vi "Queue_Driver.vi"   [LabVIEW 2023]
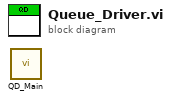
[diagram p0: block diagram]
diagram:
  n1 = call "QD_Main.vi"() -> ()  [unwired: 13 in, 3 out]
